vi "HFRR ADV v01.vi"() -> ()   [LabVIEW 2025] (continued)
                n2440 = local read "TEST STANDARD"() -> (w3160:T5)
                n2441 = Equal?(x=w3165, y=enum16{"ASTM D6079", "ISO 12156", "Custom"}."ISO 12156" ("Test Standard")) -> (x = y?=w3163:bool)
                n2442 = Equal?(x=w3160, y=enum16{"ASTM D6079", "ISO 12156", "Custom"}."ASTM D6079" ("Test Standard")) -> (x = y?=w3159:bool)
                n2443 = case shown="True" w3163 {
                  frame False {
                  }
                  frame True {
                    n2444 = local write "airtempflg"(FALSE ("airtempflg")) -> ()
                    n2445 = local write item#-1(TRUE ("Heater")) -> ()
                  }
                }
                n2446 = case shown="True" w3159 {
                  frame False {
                  }
                  frame True {
                    n2447 = local write "airtempflg"(TRUE ("airtempflg")) -> ()
                    n2448 = local write item#-1(FALSE ("Heater")) -> ()
                  }
                }
              }
            }
          }
          frame Enabled {
          }
        }
        n2449 = stacked-sequence {
          frame #0 {
            n2450 = case shown="True" "RST FF" {
              frame False {
              }
              frame True {
                w3179 = 0.0 ("X Scale.Range:Maximum")
                n2451 = property on="Frictional Force ( N )" class="WFChart (strict)"("XScale.Maximum"=600.0 ("X Scale.Range:Maximum"), "XScale.Minimum"=w3179, "YScale.Maximum"=10.0 ("Y Scale.Range:Maximum"), "YScale.Minimum"=w3179) -> ()  [unwired: 2 in, 2 out]
              }
            }
          }
          frame #1 {
            n2452 = case shown="True" "RST TEMP" {
              frame False {
              }
              frame True {
                n2453 = property on="Temperature ( Deg C )" class="WFChart (strict)"("XScale.Minimum"=0.0 ("X Scale.Range:Minimum"), "XScale.Maximum"=600.0 ("X Scale.Range:Maximum"), "YScale.Minimum"=0.0 ("Y Scale.Range:Minimum"), "YScale.Maximum"=100.0 ("Y Scale.Range:Maximum")) -> ()  [unwired: 2 in, 2 out]
              }
            }
          }
          frame #2 {
            n2454 = case shown="True" "RSTCOF" {
              frame False {
              }
              frame True {
                n2455 = property on="Coefficient of Friction" class="WFChart (strict)"("XScale.Minimum"=0.0 ("X Scale.Range:Minimum"), "XScale.Maximum"=600.0 ("X Scale.Range:Maximum"), "YScale.Maximum"=1.0 ("X Scale.Range:Minimum"), "YScale.Minimum"=0.0 ("X Scale.Range:Minimum")) -> ()  [unwired: 2 in, 2 out]
              }
            }
          }
          frame #3 {
            n2456 = case shown="True" "RSTCOF 2" {
              frame False {
              }
              frame True {
                (unwired) 100.0 ("Y Scale.Range:Maximum")
                (unwired) 0.0 ("Y Scale.Range:Minimum")
                (unwired) 600.0 ("X Scale.Range:Maximum")
                (unwired) 0.0 ("X Scale.Range:Minimum")
              }
            }
          }
          frame #4 {
            n2457 = case shown="True" "RSTCOF 3" {
              frame False {
              }
              frame True {
                n2458 = property on="Electrical Contact Resistance ( % )" class="WFChart (strict)"("XScale.Minimum"=0.0 ("X Scale.Range:Minimum"), "XScale.Maximum"=600.0 ("X Scale.Range:Maximum"), "YScale.Minimum"=0.0 ("Y Scale.Range:Minimum"), "YScale.Maximum"=100.0 ("Y Scale.Range:Maximum")) -> ()  [unwired: 2 in, 2 out]
              }
            }
          }
        }
        n2459 = local read "RUN"() -> (w3106:bool)
        n2460 = case shown="False" w3106 {
          frame False {
          }
          frame True {
          }
        }
        n2461 = local read "RUN"() -> (w3110:bool)
        n2462 = case shown="False" w3110 {
          tunnel: [FALSE ("TEST RUNNING") TRUE ("TEST RUNNING")] -> w3109
          frame False {
            w3198 = 0.0 ("Flag")
            n2463 = local write "Elapsed time"(0.0 ("elapsedtime")) -> ()
            n2464 = local write "Time Remaining"(w3198) -> ()
            n2465 = local write "Flag"(w3198) -> ()
            n2466 = local write "Remaining Time"(w3198) -> ()
          }
          frame True {
            n2467 = local write "Flag"(10.0 ("Flag")) -> ()
          }
        }
        n2468 = local read "AIR TEMP"() -> (w3104:dbl)
        n2469 = Greater Or Equal?(x=w3104, y=15.0) -> (x >= y?=w3105:bool)
        "powstat" <- w3105
        n2470 = case shown="True" "Save & Continue" {
          frame False {
          }
          frame True {
            n2471 = local read "USER ID"() -> (w3502:string)
            n2472 = local read "FILE"() -> (w3510:string)
            n2473 = String Length(string=w3510) -> (length=w3508:i32)
            n2474 = String Length(string=w3502) -> (length=w3505:i32)
            n2475 = Greater?(x=w3508, y=0) -> (0:w3507:bool)
            n2476 = Greater?(x=w3505, y=0) -> (0:w3504:bool)
            n2477 = And(x=w3507, y=w3504) -> (x .and. y?=w3503:bool)
            n2478 = case shown="True" w3503 {
              frame False {
                n2479 = stacked-sequence {
                  frame #0 {
                    n2480 = One Button Dialog(message="Please Enter a File Name and Operator ID to save data !", button name ("OK")="Ok") -> ()  [unwired: 1 out]
                  }
                  frame #1 {
                    n2481 = local write "Save & Continue"(FALSE ("OK Button")) -> ()
                  }
                }
                n2482 = local write "Save & Continue"(FALSE ("OK Button")) -> ()
              }
              frame True {
                n2483 = stacked-sequence {
                  frame #0 {
                    n2484 = local read "FILE"() -> (w3516:string)
                    n2485 = call "file check.vi"("file name in"=w3516) -> ("file name out"=w3515:string)  [unwired: 9 in, 1 out]
                    n2486 = call <vilib>:"Application Directory.vi"() -> ("Application Directory"=w3526:path)
                    n2487 = Build Path(base path=w3526, name or relative path="data") -> (appended path=w3525:path)
                    n2488 = call <vilib>:"Trim Whitespace.vi"("string"=w3515) -> ("trimmed string"=w3523:string)  [unwired: 1 in]
                    n2489 = call <vilib>:"Trim Whitespace.vi"("string"=w3515) -> ("trimmed string"=w3524:string)  [unwired: 1 in]
                    n2490 = List Folder(path=w3525) -> (folder names=w3521:string[])  [unwired: 3 in, 3 out]
                    n2491 = Match Pattern(string=w3523, regular expression="_(") -> (before substring=w3520:string)  [unwired: 1 in, 3 out]
                    n2492 = for {
                      tunnel: w3521 -> [w3535] mode=indexing
                      tunnel: w3520 -> [w3533]
                      shift-right: [w3531] -> w3518
                      shift-left: bool[] [] -> [w3532]
                      n2493 = Match Pattern(string=w3535, regular expression="_(") -> (before substring=w3534:string)  [unwired: 1 in, 3 out]
                      n2494 = Equal?(x=w3534, y=w3533) -> (x = y?=w3530:bool)
                      n2495 = case shown="True" w3530 {
                        tunnel: w3530 -> [_ w3538]
                        tunnel: w3532 -> [w3537 w3540]
                        tunnel: [w3537 w3539] -> w3531
                        frame False {
                        }
                        frame True {
                          n2496 = Insert Into Array(array=w3540, new element=w3538) -> (w3539:bool[])  [unwired: 1 in]
                        }
                      }
                    }
                    n2497 = Equal?(x=w3521, y=w3520) -> (x = y?=w3529:bool[])
                    n2498 = Or Array Elements(Boolean array=w3529) -> (logical OR=w3528:bool)
                    n2499 = Array Size(array=w3518) -> (size(s)=w3517:i32)
                    n2500 = case shown="True" w3528 {
                      tunnel: w3524 -> [_ w3548]
                      tunnel: w3517 -> [_ w3541]
                      frame False {
                      }
                      frame True {
                        n2501 = Number To Decimal String(number=w3541) -> (decimal integer string=w3544:string)  [unwired: 1 in]
                        n2502 = Search/Split String(string=w3548, search string/char (-)="_(" ("regular expression")) -> (substring before match=w3546:string)  [unwired: 1 in, 2 out]
                        n2503 = Concatenate Strings(w3546, "_(" ("regular expression"), w3544, ")" ("regular expression")) -> (w3542:string)
                        n2504 = local write "FILE"(w3542) -> ()
                      }
                    }
                  }
                  frame #1 {
                    w3551 = 0.0
                    w3564 = cluster{"y":dbl, dbl, "y":dbl}[] [] ("History Data")
                    w3565 = FALSE ("Heater Button")
                    (unwired) ")!" ("string")
                    (unwired) ")" ("string")
                    w3563 = dbl[] [] ("History Data")
                    w3569 = "\r"
                    # "C:\\WinDucom\\Data\\"
                    # "C:\\LAB-IQ-NXT\\data"
                    n2505 = local write "Humidity ( %RH )"(w3551) -> ()
                    n2506 = local write "Frequency ( Hz )"(w3551) -> ()
                    n2507 = local write "Stroke 3"(w3551) -> ()
                    n2508 = local write "speedop"(0.0 ("PIDclk 2")) -> ()
                    n2509 = local write "Set Temp 2"(65.0 ("Set Temp 2")) -> ()
                    n2510 = local write "AIR TEMP"(w3551) -> ()
                    n2511 = local write "clk"(0.0 ("clk")) -> ()
                    n2512 = local write "Stroke 4"(w3551) -> ()
                    n2513 = local write "COF 2"(w3551) -> ()
                    n2514 = local write "TEMP"(w3551) -> ()
                    n2515 = local write "ecr 3"(w3551) -> ()
                    n2516 = local write "FF 3"(w3551) -> ()
                    n2517 = local write "FF 2"(w3551) -> ()
                    n2518 = property on="Coefficient of Friction" class="WFChart (strict)"("History Data"=w3563) -> ()  [unwired: 2 in, 2 out]
                    n2519 = property on="Coefficient of Friction" class="WFChart (strict)"("History Data"=w3563) -> ()  [unwired: 2 in, 2 out]
                    n2520 = property on="Frictional Force ( N )" class="WFChart (strict)"("History Data"=w3563) -> ()  [unwired: 2 in, 2 out]
                    n2521 = property on="Electrical Contact Resistance ( % )" class="WFChart (strict)"("History Data"=w3563) -> ()  [unwired: 2 in, 2 out]
                    n2522 = property on="Electrical Contact Resistance ( % )" class="WFChart (strict)"("History Data"=w3563) -> ()  [unwired: 2 in, 2 out]
                    n2523 = property on="Temperature ( Deg C )" class="WFChart (strict)"("History Data"=w3563) -> ()  [unwired: 2 in, 2 out]
                    n2524 = property on="Frictional Force ( N )" class="WFChart (strict)"("History Data"=w3563) -> ()  [unwired: 2 in, 2 out]
                    n2525 = property on="Coefficient of Friction" class="WFChart (strict)"("History Data"=w3563) -> ()  [unwired: 2 in, 2 out]
                    n2526 = property on="Frictional Force ( N )" class="WFChart (strict)"("History Data"=w3563) -> ()  [unwired: 2 in, 2 out]
                    n2527 = property on="Electrical Contact Resistance ( % )" class="WFChart (strict)"("History Data"=w3563) -> ()  [unwired: 2 in, 2 out]
                    n2528 = property on="Temperature ( Deg C )" class="WFChart (strict)"("History Data"=w3563) -> ()  [unwired: 2 in, 2 out]
                    n2529 = property on="Stroke ( mm )" class="WFChart (strict)"("History Data"=w3564) -> ()  [unwired: 2 in, 2 out]
                    n2530 = property on="Stroke ( mm )" class="WFChart (strict)"("History Data"=w3564) -> ()  [unwired: 2 in, 2 out]
                    n2531 = local write "Humidity"(w3565) -> ()
                    n2532 = local write "Heater Button"(w3565) -> ()
                    n2533 = local read "FILE"() -> (w3559:string)
                    n2534 = disable-structure shown="Enabled" {
                      disable-tunnel: [w3603 _] -> w3550
                      frame Enabled {
                        n2535 = local read "NORMAL LOAD"() -> (w3603:dbl)
                      }
                      frame Disabled {
                      }
                    }
                    n2536 = call "file check.vi"("file name in"=w3559) -> ("error out"=w3562:errorcluster, "file name out"=w3556:string)  [unwired: 9 in]
                    n2537 = call "FILE PATH CREATION.vi"("error in"=w3562, "FILE NAME :"=w3556) -> ("FILE OUT"=w3555:path)  [unwired: 8 in, 1 out]
                    n2538 = Concatenate Strings(w3556, ".dgf" ("Substring")) -> (w3561:string)
                    n2539 = Concatenate Strings(w3556, ".duf" ("Substring")) -> (w3557:string)
                    n2540 = Multiply(x=w3550, y=1.0) -> (x*y=w3582:dbl)
                    n2541 = Build Path(base path=w3555, name or relative path=w3561) -> (appended path=w3554:path)
                    n2542 = Build Path(base path=w3555, name or relative path=w3557) -> (appended path=w3553:path)
                    n2543 = Number To Fractional String(number=w3582, width (-)=i16 5, precision (6)=i16 2) -> (F-format string=w3590:string)  [unwired: 1 in]
                    n2544 = local read "tested by"() -> (w3549:string)
                    n2545 = local read "Fuel Discription :"() -> (w3578:string)
                    n2546 = local read "Batch Ref Num :"() -> (w3567:string)
                    n2547 = Get Date/Time String(date format (0)=enum16{"short", "long", "abbreviated"}."short") -> (date string=w3601:string, time string=w3598:string)  [unwired: 2 in]
                    n2548 = local read "Remarks :"() -> (w3577:string)
                    n2549 = Concatenate Strings("Load :- " ("Substring"), w3590, " grams ," ("Substring")) -> (w3589:string)
                    n2550 = local read "String 41"() -> (w3570:string)
                    n2551 = Concatenate Strings(w3578) -> (w3579:string)
                    n2552 = Concatenate Strings(w3567) -> (w3566:string)
                    n2553 = Concatenate Strings(w3549) -> (w3573:string)
                    n2554 = Concatenate Strings("(" ("Substring"), w3601, ")" ("Substring"), w3598) -> (w3572:string)
                    "concatenated string" <- w3572
                    n2555 = Concatenate Strings(w3577, "," ("string")) -> (w3576:string)
                    n2556 = Concatenate Strings("  TIME;      COF;       STROKE;     AIR TEMP;  TEMP;  HUMIDITY;  ECR; PID-OUT; FREQUENCY" ("Substring"), "\r") -> (w3585:string)
                    n2557 = Concatenate Strings(w3570, w3569, "Fuel Discription :-" ("Substring"), w3579, w3569, w3589, w3569, "Batch Ref Num :-" ("Substring"), w3566, w3569, " Remarks :- " ("Substring"), w3576, w3569, " Date :- " ("Substring"), w3572, w3569, "Tested By :-" ("Substring"), w3573) -> (w3583:string)
                    "REMARKS" <- w3583
                    n2558 = call <vilib>:"Write Characters To File.vi"("append to file? (new file:F)"=FALSE, "character string"=w3585, "file path (dialog if empty)"=w3554) -> ()  [unwired: 2 in, 1 out]
                    n2559 = call <vilib>:"Write Characters To File.vi"("append to file? (new file:F)"=FALSE, "character string"=w3583, "file path (dialog if empty)"=w3553) -> ()  [unwired: 2 in, 1 out]
                  }
                  frame #2 {
                    n2560 = local write "Cycles elapsed"(0 ("Cycles elapsed")) -> ()
                    n2561 = local write "cyclecount"(0 ("cyclecount")) -> ()
                    n2562 = local write "Save & Continue"(FALSE ("OK")) -> ()
                    n2563 = local write "autostrtflg"(TRUE ("autostrtflg")) -> ()
                    n2564 = local write "Save"(FALSE ("Save")) -> ()
                    n2565 = Get Date/Time In Seconds() -> (seconds since 1Jan1904=w3608:timestamp)
                    n2566 = To Double Precision Float(number=w3608) -> (double precision float=w3607:dbl)
                    n2567 = local write "acq timer"(w3607) -> ()
                    n2568 = One Button Dialog(message="Please ensure sample is mounted properly and machine is ready in all aspects for testing !", button name ("OK")="Ok") -> ()  [unwired: 1 out]
                  }
                  frame #3 {
                    n2569 = stacked-sequence {
                      frame #0 {
                        n2570 = local write "Main Dashboard Buttons"(T1."Dashboard" ("Main Dashboard Buttons")) -> ()
                        n2571 = local write "Main Tab"(T4."Acquire" ("Main Tab")) -> ()
                      }
                      frame #1 {
                        n2572 = local write "EVENT LOG"("" ("EVENT LOG")) -> ()
                      }
                      frame #2 {
                        n2573 = Wait (ms)(milliseconds to wait=u32 50) -> ()  [unwired: 1 out]
                      }
                      frame #3 {
                        n2574 = disable-structure shown="Disabled" {
                          frame Disabled {
                            n2575 = local read "EVENT LOG"() -> (w3620:string)
                            n2576 = call "Event Log.vi"("Content"="Test Details", "EVENT LOG"=w3620) -> ("EVENT LOG"=w3619:string)  [unwired: 8 in, 1 out]
                            n2577 = local write "EVENT LOG"(w3619) -> ()
                          }
                          frame Enabled {
                          }
                        }
                      }
                      frame #4 {
                        n2578 = Wait (ms)(milliseconds to wait=u32 50) -> ()  [unwired: 1 out]
                      }
                      frame #5 {
                        n2579 = local read "FILE"() -> (w3622:string)
                        n2580 = Concatenate Strings("File Name :" ("Content"), w3622) -> (w3623:string)
                        n2581 = local read "EVENT LOG"() -> (w3626:string)
                        n2582 = call "Event Log.vi"("Content"=w3623, "EVENT LOG"=w3626) -> ("EVENT LOG"=w3625:string)  [unwired: 8 in, 1 out]
                        n2583 = local write "EVENT LOG"(w3625) -> ()
                      }
                      frame #6 {
                        n2584 = Wait (ms)(milliseconds to wait=u32 50) -> ()  [unwired: 1 out]
                      }
                      frame #7 {
                        n2585 = local read "Batch Ref Num :"() -> (w3628:string)
                        n2586 = Concatenate Strings("Batch Ref No :" ("Content"), w3628) -> (w3629:string)
                        n2587 = local read "EVENT LOG"() -> (w3632:string)
                        n2588 = call "Event Log.vi"("Content"=w3629, "EVENT LOG"=w3632) -> ("EVENT LOG"=w3631:string)  [unwired: 8 in, 1 out]
                        n2589 = local write "EVENT LOG"(w3631) -> ()
                      }
                      frame #8 {
                        n2590 = Wait (ms)(milliseconds to wait=u32 50) -> ()  [unwired: 1 out]
                      }
                      frame #9 {
                        n2591 = local read "tested by"() -> (w3634:string)
                        n2592 = Concatenate Strings("Tested By :" ("Content"), w3634) -> (w3635:string)
                        n2593 = local read "EVENT LOG"() -> (w3638:string)
                        n2594 = call "Event Log.vi"("Content"=w3635, "EVENT LOG"=w3638) -> ("EVENT LOG"=w3637:string)  [unwired: 8 in, 1 out]
                        n2595 = local write "EVENT LOG"(w3637) -> ()
                      }
                      frame #10 {
                        n2596 = Wait (ms)(milliseconds to wait=u32 50) -> ()  [unwired: 1 out]
                      }
                      frame #11 {
                        n2597 = local read "TEST STANDARD"() -> (w3641:T5)
                        n2598 = case shown="\"ASTM D6079\", Default" w3641 {
                          tunnel: ["ASTM D6079" "ISO 12156" "CEC F-096-A-06" "Custom"] -> w3640
                          frame "ASTM D6079", Default {
                          }
                          frame "ISO 12156" {
                          }
                          frame "CEC F-096-A-06" {
                          }
                          frame "Custom" {
                          }
                        }
                        n2599 = Concatenate Strings("Test Standard :" ("Content"), w3640) -> (w3642:string)
                        n2600 = local read "EVENT LOG"() -> (w3645:string)
                        n2601 = call "Event Log.vi"("Content"=w3642, "EVENT LOG"=w3645) -> ("EVENT LOG"=w3644:string)  [unwired: 8 in, 1 out]
                        n2602 = local write "EVENT LOG"(w3644) -> ()
                      }
                      frame #12 {
                        n2603 = Wait (ms)(milliseconds to wait=u32 50) -> ()  [unwired: 1 out]
                      }
                      frame #13 {
                        n2604 = local read "Fuel Discription :"() -> (w3651:string)
                        n2605 = Concatenate Strings("Fuel Description :" ("Content"), w3651) -> (w3652:string)
                        n2606 = local read "EVENT LOG"() -> (w3655:string)
                        n2607 = call "Event Log.vi"("Content"=w3652, "EVENT LOG"=w3655) -> ("EVENT LOG"=w3654:string)  [unwired: 8 in, 1 out]
                        n2608 = local write "EVENT LOG"(w3654) -> ()
                      }
                      frame #14 {
                        n2609 = Wait (ms)(milliseconds to wait=u32 50) -> ()  [unwired: 1 out]
                      }
                      frame #15 {
                        n2610 = local read "Remarks :"() -> (w3657:string)
                        n2611 = Concatenate Strings("Remarks :" ("Content"), w3657) -> (w3658:string)
                        n2612 = local read "EVENT LOG"() -> (w3661:string)
                        n2613 = call "Event Log.vi"("Content"=w3658, "EVENT LOG"=w3661) -> ("EVENT LOG"=w3660:string)  [unwired: 8 in, 1 out]
                        n2614 = local write "EVENT LOG"(w3660) -> ()
                      }
                      frame #16 {
                        n2615 = Wait (ms)(milliseconds to wait=u32 50) -> ()  [unwired: 1 out]
                      }
                      frame #17 {
                        n2616 = local read "USER ID"() -> (w3663:string)
                        n2617 = Concatenate Strings("Operator ID :" ("Content"), w3663) -> (w3665:string)
                        n2618 = local read "EVENT LOG"() -> (w3667:string)
                        n2619 = call "Event Log.vi"("Content"=w3665, "EVENT LOG"=w3667) -> ("EVENT LOG"=w3666:string)  [unwired: 8 in, 1 out]
                        n2620 = local write "EVENT LOG"(w3666) -> ()
                      }
                      frame #18 {
                        n2621 = Wait (ms)(milliseconds to wait=u32 50) -> ()  [unwired: 1 out]
                      }
                      frame #19 {
                        n2622 = disable-structure shown="Disabled" {
                          frame Disabled {
                            n2623 = local read "EVENT LOG"() -> (w3671:string)
                            n2624 = call "Event Log.vi"("Content"="Test Parameter", "EVENT LOG"=w3671) -> ("EVENT LOG"=w3670:string)  [unwired: 8 in, 1 out]
                            n2625 = local write "EVENT LOG"(w3670) -> ()
                          }
                          frame Enabled {
                          }
                        }
                      }
                      frame #20 {
                        n2626 = Wait (ms)(milliseconds to wait=u32 50) -> ()  [unwired: 1 out]
                      }
                      frame #21 {
                        n2627 = local read "Set Hz"() -> (w3675:dbl)
                        n2628 = Number To Fractional String(number=w3675, precision (6)=i16 2) -> (F-format string=w3674:string)  [unwired: 2 in]
                        n2629 = Concatenate Strings("Set Frequency [Hz] :" ("Content"), w3674) -> (w3677:string)
                        n2630 = local read "EVENT LOG"() -> (w3679:string)
                        n2631 = call "Event Log.vi"("Content"=w3677, "EVENT LOG"=w3679) -> ("EVENT LOG"=w3678:string)  [unwired: 8 in, 1 out]
                        n2632 = local write "EVENT LOG"(w3678) -> ()
                      }
                      frame #22 {
                        n2633 = Wait (ms)(milliseconds to wait=u32 50) -> ()  [unwired: 1 out]
                      }
                      frame #23 {
                        n2634 = local read "NORMAL LOAD"() -> (w3682:dbl)
                        n2635 = Number To Fractional String(number=w3682, precision (6)=i16 2) -> (F-format string=w3683:string)  [unwired: 2 in]
                        n2636 = Concatenate Strings("Applied Load [grams] :" ("Content"), w3683) -> (w3685:string)
                        n2637 = local read "EVENT LOG"() -> (w3687:string)
                        n2638 = call "Event Log.vi"("Content"=w3685, "EVENT LOG"=w3687) -> ("EVENT LOG"=w3686:string)  [unwired: 8 in, 1 out]
                        n2639 = local write "EVENT LOG"(w3686) -> ()
                      }
                      frame #24 {
                        n2640 = Wait (ms)(milliseconds to wait=u32 50) -> ()  [unwired: 1 out]
                      }
                      frame #25 {
                        n2641 = local read "Set Strk"() -> (w3690:dbl)
                        n2642 = Number To Fractional String(number=w3690, precision (6)=i16 2) -> (F-format string=w3691:string)  [unwired: 2 in]
                        n2643 = Concatenate Strings("Set Stroke [mm] :" ("Content"), w3691) -> (w3693:string)
                        n2644 = local read "EVENT LOG"() -> (w3695:string)
                        n2645 = call "Event Log.vi"("Content"=w3693, "EVENT LOG"=w3695) -> ("EVENT LOG"=w3694:string)  [unwired: 8 in, 1 out]
                        n2646 = local write "EVENT LOG"(w3694) -> ()
                      }
                      frame #26 {
                        n2647 = Wait (ms)(milliseconds to wait=u32 50) -> ()  [unwired: 1 out]
                      }
                      frame #27 {
                        n2648 = local read "Set Temp"() -> (w3698:dbl)
                        n2649 = Number To Fractional String(number=w3698, precision (6)=i16 2) -> (F-format string=w3699:string)  [unwired: 2 in]
                        n2650 = Concatenate Strings("Set Temperature [deg C] :" ("Content"), w3699) -> (w3701:string)
                        n2651 = local read "EVENT LOG"() -> (w3703:string)
                        n2652 = call "Event Log.vi"("Content"=w3701, "EVENT LOG"=w3703) -> ("EVENT LOG"=w3702:string)  [unwired: 8 in, 1 out]
                        n2653 = local write "EVENT LOG"(w3702) -> ()
                      }
                      frame #28 {
                        n2654 = Wait (ms)(milliseconds to wait=u32 50) -> ()  [unwired: 1 out]
                      }
                      frame #29 {
                        n2655 = local read "Set Rh"() -> (w3706:dbl)
                        n2656 = Number To Fractional String(number=w3706, precision (6)=i16 2) -> (F-format string=w3707:string)  [unwired: 2 in]
                        n2657 = Concatenate Strings("Set Humidity [%RH] :" ("Content"), w3707) -> (w3709:string)
                        n2658 = local read "EVENT LOG"() -> (w3711:string)
                        n2659 = call "Event Log.vi"("Content"=w3709, "EVENT LOG"=w3711) -> ("EVENT LOG"=w3710:string)  [unwired: 8 in, 1 out]
                        n2660 = local write "EVENT LOG"(w3710) -> ()
                      }
                      frame #30 {
                        n2661 = Wait (ms)(milliseconds to wait=u32 50) -> ()  [unwired: 1 out]
                      }
                      frame #31 {
                        n2662 = local read "test time"() -> (w3714:dbl)
                        n2663 = Number To Fractional String(number=w3714, precision (6)=i16 1) -> (F-format string=w3715:string)  [unwired: 2 in]
                        n2664 = Concatenate Strings("Test Duration [mins] :" ("Content"), w3715) -> (w3717:string)
                        n2665 = local read "EVENT LOG"() -> (w3719:string)
                        n2666 = call "Event Log.vi"("Content"=w3717, "EVENT LOG"=w3719) -> ("EVENT LOG"=w3718:string)  [unwired: 8 in, 1 out]
                        n2667 = local write "EVENT LOG"(w3718) -> ()
                      }
                      frame #32 {
                        w3720 = dbl[] [] ("History Data")
                        w3721 = cluster{"y":dbl, dbl, "y":dbl}[] [] ("History Data")
                        w3722 = FALSE ("Visible")
                        n2668 = property on="Stroke ( mm )" class="WFChart (strict)"("History Data"=w3721) -> ()  [unwired: 2 in, 2 out]
                        n2669 = property on="Temperature ( Deg C )" class="WFChart (strict)"("History Data"=w3720) -> ()  [unwired: 2 in, 2 out]
                        n2670 = property on="Electrical Contact Resistance ( % )" class="WFChart (strict)"("History Data"=w3720) -> ()  [unwired: 2 in, 2 out]
                        n2671 = property on="Coefficient of Friction" class="WFChart (strict)"("History Data"=w3720) -> ()  [unwired: 2 in, 2 out]
                        n2672 = property on="Frictional Force ( N )" class="WFChart (strict)"("History Data"=w3720) -> ()  [unwired: 2 in, 2 out]
                        n2673 = property on="Coefficient of Friction" class="WFChart (strict)"("History Data"=w3720) -> ()  [unwired: 2 in, 2 out]
                        n2674 = property on="Frictional Force ( N )" class="WFChart (strict)"("History Data"=w3720) -> ()  [unwired: 2 in, 2 out]
                        n2675 = property on="Electrical Contact Resistance ( % )" class="WFChart (strict)"("History Data"=w3720) -> ()  [unwired: 2 in, 2 out]
                        n2676 = property on="Stroke ( mm )" class="WFChart (strict)"("History Data"=w3721) -> ()  [unwired: 2 in, 2 out]
                        n2677 = property on="Temperature ( Deg C )" class="WFChart (strict)"("History Data"=w3720) -> ()  [unwired: 2 in, 2 out]
                        n2678 = property on="Service Password Log" class="Str"("Visible"=w3722) -> ()  [unwired: 2 in, 2 out]
                        n2679 = property on="Password 3" class="Clust (strict)"("Visible"=w3722) -> ()  [unwired: 2 in, 2 out]
                      }
                    }
                    "TEST FILE NAM,E SAVED" <- TRUE ("TEST FILE NAM,E SAVED")
                  }
                }
              }
            }
          }
        }
        n2680 = local write "Test \nStatus"(w3109) -> ()
        n2681 = local write "Save"(w3109) -> ()
        n2682 = local read "Main Tab"() -> (w3103:T4)
        n2683 = case shown="True" w3106 {
          frame False {
            n2684 = local read "Rt 3"() -> (w3170:bool)
            n2685 = case shown="True" w3170 {
              frame False {
              }
              frame True {
                n2686 = local write "Rt 3"(FALSE ("Rt 3")) -> ()
              }
            }
            "Rt" <- TRUE ("Rt")
            "Rt 2" <- FALSE ("Rt")
          }
          frame True {
            n2687 = local read "Rt"() -> (w3176:bool)
            n2688 = local write "Rt 2"(TRUE ("Rt 2")) -> ()
            n2689 = case shown="True" w3176 {
              frame False {
              }
              frame True {
                n2690 = local write "Rt"(FALSE ("Rt")) -> ()
              }
            }
            "Rt 3" <- TRUE ("Rt 3")
          }
        }
        n2691 = case shown="\"Acquire\"" w3103 {
          tunnel: w3105 -> [_ w3205]
          frame Default {
            w3204 = 0.0 ("output")
            n2692 = local write "PID-out"(w3204) -> ()
            n2693 = local write "Frequency ( Hz )"(w3204) -> ()
            n2694 = local write "STROKE Initialize"(TRUE ("STROKE Initialize")) -> ()
          }
          frame "Acquire" {
            n2695 = stacked-sequence {
              frame #0 {
                n2696 = local read "Auto Start Test"() -> (w3207:bool)
                n2697 = case shown="True" w3207 {
                  tunnel: "RUN" -> [w3228 w3231]
                  tunnel: [w3228 w3230] -> w3208
                  frame False {
                  }
                  frame True {
                    n2698 = local read "Auto Start Temp"() -> (w3229:bool)
                    n2699 = Or(x=w3231, y=w3229) -> (x .or. y?=w3230:bool)
                  }
                }
                n2700 = local read "clk"() -> (w3227:dbl)
                n2701 = local read "Save"() -> (w3223:bool)
                n2702 = Equal?(x=w3227, y=0.0) -> (x = y?=w3224:bool)
                n2703 = And(x=w3224, y=w3223) -> (x .and. y?=w3225:bool)
                n2704 = Not(x="Engage") -> (.not. x?=w3214:bool)
                n2705 = case shown="False" w3208 {
                  tunnel: [0.0 w3255] -> w3210
                  frame False {
                    (unwired) TRUE ("Visible")
                    n2706 = local read "Auto Start Test"() -> (w3235:bool)
                    n2707 = local write "Start Time"(TRUE ("Start Time")) -> ()
                    n2708 = property on="Stroke 2" class="DigNum (strict)"("Visible"=FALSE) -> ()  [unwired: 2 in, 2 out]
                    n2709 = case shown="False" w3235 {
                      frame False {
                        n2710 = property on="Heater Button" class="Bool (strict)"("DisabledEnum"=T19."Enabled" ("Disabled")) -> ()  [unwired: 2 in, 2 out]
                        n2711 = property on="Humidity" class="Bool (strict)"("DisabledEnum"=T19."Enabled" ("Disabled")) -> ()  [unwired: 2 in, 2 out]
                      }
                      frame True {
                      }
                    }
                    n2712 = case shown="False" "TestCompFlg" {
                      frame False {
                        n2713 = local read "StartFlg"() -> (w3243:bool)
                        n2714 = case shown="True" w3243 {
                          frame False {
                          }
                          frame True {
                            n2715 = stacked-sequence {
                              frame #0 {
                                n2716 = local read "EVENT LOG"() -> (w3247:string)
                                n2717 = call "Event Log.vi"("Content"="Test was interrupted", "EVENT LOG"=w3247) -> ("EVENT LOG"=w3248:string)  [unwired: 8 in, 1 out]
                                n2718 = local write "EVENT LOG"(w3248) -> ()
                                n2719 = property on="RUN" class="Bool (strict)"("Visible"=TRUE) -> ()  [unwired: 2 in, 2 out]
                                n2720 = property on="Auto Start Test" class="Bool (strict)"("Visible"=TRUE) -> ()  [unwired: 2 in, 2 out]
                              }
                              frame #1 {
                                w3251 = FALSE ("StartFlg")
                                n2721 = property on="Heater Button" class="Bool (strict)"("Val(Sgnl)"=FALSE ("Value (Signaling)")) -> ()  [unwired: 2 in, 2 out]
                                n2722 = local write "Heater Button"(w3251) -> ()
                                n2723 = local write "StartFlg"(w3251) -> ()
                                n2724 = local write "Humidity"(w3251) -> ()
                                n2725 = local write "Humidity 2"(TRUE ("Humidity")) -> ()
                              }
                              frame #2 {
                                n2726 = local write "Due Write"("VC;0" ("Command")) -> ()
                              }
                              frame #3 {
                                n2727 = Wait (ms)(milliseconds to wait=u32 1500) -> ()  [unwired: 1 out]
                              }
                              frame #4 {
                                n2728 = local write "Due Write"("HE;0" ("Command")) -> ()
                              }
                            }
                          }
                        }
                      }
                      frame True {
                      }
                    }
                    n2729 = local write "String 14"("Test will autostart once parameters reach the set value." ("String 14")) -> ()
                  }
                  frame True {
                    (unwired) FALSE ("Visible")
                    n2730 = property on="Stroke 2" class="DigNum (strict)"("Visible"=TRUE) -> ()  [unwired: 2 in, 2 out]
                    n2731 = property on="STOP 2" class="Bool (strict)"("Disabled"=u8 2) -> ()  [unwired: 2 in, 2 out]
                    n2732 = local write "String 14"(" Running....." ("String 14")) -> ()
                    n2733 = property on="Heater Button" class="Bool (strict)"("DisabledEnum"=T19."Disabled and Grayed Out" ("Disabled")) -> ()  [unwired: 2 in, 2 out]
                    n2734 = property on="Humidity" class="Bool (strict)"("DisabledEnum"=T19."Disabled and Grayed Out" ("Disabled")) -> ()  [unwired: 2 in, 2 out]
                    n2735 = case shown="True" "Start Time" {
                      selector: "Start Time" -> [_ w3274]
                      frame False {
                      }
                      frame True {
                        n2736 = Not(x=w3274) -> (.not. x?=w3273:bool)
                        n2737 = local write "Start Time"(w3273) -> ()
                        n2738 = local read "EVENT LOG"() -> (w3275:string)
                        n2739 = call "Event Log.vi"("Content"="Test in progress", "EVENT LOG"=w3275) -> ("EVENT LOG"=w3277:string)  [unwired: 8 in, 1 out]
                        n2740 = local write "EVENT LOG"(w3277) -> ()
                      }
                    }
                    n2741 = disable-structure shown="Enabled" {
                      disable-tunnel: [w3266 w3272] -> w3255
                      frame Disabled {
                        n2742 = local read "Set Hz"() -> (w3269:dbl)
                        n2743 = call <vilib>:"Uniform White Noise Waveform.vi"() -> ("signal out"=w3268:waveform(dbl))  [unwired: 10 in, 1 out]
                        n2744 = Random Number (0-1)() -> (number: 0 to 1=w3265:dbl)
                        n2745 = Add(x=w3269, y=w3268) -> (x+y=w3267:waveform(dbl))
                        n2746 = Multiply(x=ext 0.01 ("y"), y=w3265) -> (x*y=w3263:ext)
                        n2747 = Multiply(x=w3267, y=w3263) -> (x*y=w3266:waveform(ext))
                      }
                      frame Enabled {
                        n2748 = call-poly <vilib>:"Random Number (Range).vi"("lower bound (0)"=49.89, "upper bound (100)"=50.8) -> ("number"=w3272:dbl)  [unwired: 9 in]
                      }
                    }
                    "StartFlg" <- TRUE ("StartFlg")
                  }
                }
                n2749 = case shown="True" w3225 {
                  frame False {
                  }
                  frame True {
                    n2750 = local write "clk"(10.0 ("clk")) -> ()
                    n2751 = Get Date/Time In Seconds() -> (seconds since 1Jan1904=w3280:timestamp)
                    n2752 = To Double Precision Float(number=w3280) -> (double precision float=w3278:dbl)
                    n2753 = local write "acq timer"(w3278) -> ()
                    n2754 = local write "act save time"(w3278) -> ()
                  }
                }
                n2755 = call "Elapsed Time"("Time Target (s)"="Countdown", "Reset"=w3214) -> ("Elapsed Time (s)"=w3219:dbl, "Time has Elapsed"=w3217:bool)  [unwired: 10 in, 6 out]
                "Countdown 2" <- w3219
                n2756 = Subtract(x=w3219, y=2.0) -> (x-y=w3222:dbl)
                n2757 = Less?(x=w3222, y="Countdown") -> (x < y?=w3220:bool)
                n2758 = And(x=w3220, y=w3217) -> (x .and. y?=w3216:bool)
                n2759 = case shown="True" w3216 {
                  frame False {
                  }
                  frame True {
                    (unwired) dbl[] [] ("History Data")
                    n2760 = local write "Engage"(FALSE ("Engage")) -> ()
                    n2761 = local write "RUN"(TRUE ("RUN")) -> ()
                    n2762 = local read "Humidity ( %RH )"() -> (→"Rh Before":dbl)
                  }
                }
                n2763 = local read "Test \nStatus"() -> (w3212:bool)
                n2764 = Select(t=w3210, s=w3212, f=0.0) -> (s? t:f=w3211:dbl)
                n2765 = local write "Frequency ( Hz )"(w3211) -> ()
              }
              frame #1 {
                w3303 = 1000000.0 ("x")
                # "HC;1/0\nST;VALUE"
                # "Elapsed time\ncof\nstroke\nAir temp\nTemp\nHumidity"
                # "acq timer\n\nact save time"
                # "convert to microseconds"
                n2766 = local read "COUNT"() -> (w3286:i32)
                n2767 = local read "Rate"() -> (w3299:dbl)
                n2768 = Divide(x=w3303, y=w3299) -> (x/y=w3304:dbl)
                n2769 = Greater Or Equal?(x=w3286, y=250) -> (x >= y?=w3285:bool)
                n2770 = Get Date/Time In Seconds() -> (seconds since 1Jan1904=w3306:timestamp)
                n2771 = case shown="True" w3285 {
                  frame False {
                    n2772 = local read "COUNT"() -> (w3307:i32)
                    n2773 = Increment(x=w3307) -> (x+1=w3308:i32)
                    n2774 = local write "COUNT"(w3308) -> ()
                  }
                  frame True {
                    n2775 = local write "COUNT"(0 ("COUNT")) -> ()
                  }
                }
                n2776 = local read "Samplingtime 2"() -> (w3284:dbl)
                n2777 = local read "act save time"() -> (w3301:dbl)
                n2778 = Divide(x=w3304, y=w3303) -> (x/y=w3302:dbl)
                n2779 = To Double Precision Float(number=w3306) -> (double precision float=w3295:dbl)
                n2780 = Add(x=w3301, y=w3284) -> (x+y=w3300:dbl)
                n2781 = local read "acq timer"() -> (w3305:dbl)
                n2782 = local read "COUNT"() -> (w3288:i32)
                n2783 = Greater Or Equal?(x=w3295, y=w3300) -> (x >= y?=w3283:bool)
                n2784 = Multiply(x=w3302, y=w3288) -> (x*y=w3294:dbl)
                n2785 = Subtract(x=w3295, y=w3305) -> (x-y=w3297:dbl)
                n2786 = local read "Save"() -> (w3298:bool)
                n2787 = Add(x=w3297, y=w3294) -> (x+y=w3281:dbl)
                "Elapsed time 3" <- w3281
                n2788 = And(x=w3283, y=w3298) -> (x .and. y?=w3296:bool)
                n2789 = Divide(x=w3281, y=60.0) -> (x/y=w3292:dbl)
                n2790 = local read "Test \nStatus"() -> (w3282:bool)
                n2791 = local read "clk"() -> (w3289:dbl)
                n2792 = Equal?(x=w3289, y=10.0) -> (x = y?=w3291:bool)
                n2793 = case shown="True" w3296 {
                  tunnel: w3295 -> [_ w3422]
                  tunnel: [FALSE ("Boolean 2") TRUE ("Boolean 2")] -> _
                  frame False {
                  }
                  frame True {
                    w3376 = ";" ("Substring")
                    # "Pid out/\nFreq response value"
                    n2794 = local write "act save time"(w3422) -> ()
                    n2795 = local read "FILE"() -> (w3370:string)
                    n2796 = call "file check.vi"("file name in"=w3370) -> ("error out"=w3373:errorcluster, "file name out"=w3368:string)  [unwired: 9 in]
                    n2797 = local read "LVDT STROKE"() -> (w3365:dbl)
                    n2798 = local read "Add up Stroke"() -> (w3363:dbl)
                    n2799 = call "FILE PATH CREATION.vi"("error in"=w3373, "FILE NAME :"=w3368) -> ("FILE OUT"=w3371:path)  [unwired: 8 in, 1 out]
                    n2800 = local read "STROKE Initialize"() -> (w3358:bool)
                    n2801 = Concatenate Strings(w3368, ".dgf" ("Substring")) -> (w3372:string)
                    n2802 = Subtract(x=w3365, y=w3363) -> (x-y=w3364:dbl)
                    n2803 = Absolute Value(x=w3364) -> (abs(x)=w3361:dbl)
                    n2804 = local read "FF 2"() -> (→"Frictional Force ( N )" →"Frictional Force ( N )":dbl)
                    n2805 = Build Path(base path=w3371, name or relative path=w3372) -> (appended path=w3367:path)
                    n2806 = flat-sequence {
                      tunnel: w3361 -> [w3427]
                      tunnel: [w3426] -> w3359
                      tunnel: w3358 -> [w3424]
                      tunnel: [w3429] -> w3360
                      tunnel: w3359 -> [w3429]
                      frame #0 {
                        n2807 = call <vilib>:"Mean PtByPt.vi"("x"=w3427, "sample length"="STROKE FILTER", "initialize"=w3424) -> ("mean"=w3426:dbl)  [unwired: 1 in, 1 out]
                      }
                      frame #1 {
                        "STROKE Initialize" <- FALSE ("STROKE Initialize")
                      }
                    }
                    n2808 = local read "COF 2"() -> (w3381:dbl)
                    "Coefficient of Friction" <- w3381
                    "COF 4" <- w3381
                    "Coefficient of Friction" <- w3381
                    n2809 = local read "TEMP"() -> (w3384:dbl)
                    "Temperature ( Deg C )" <- w3384
                    n2810 = local read "Humidity ( %RH )"() -> (w3383:dbl)
                    n2811 = local read "Frequency ( Hz )"() -> (w3390:dbl)
                    n2812 = local read "LVDT STROKE DISPLAY"() -> (w3362:dbl)
                    n2813 = local read "Elapsed time"() -> (w3415:dbl)
                    n2814 = local read "AIR TEMP"() -> (w3388:dbl)
                    n2815 = local read "PID-out"() -> (w3393:dbl)
                    n2816 = local write "Temperature ( Deg C )"(w3384) -> ()
                    n2817 = Number To Fractional String(number=w3362, width (-)=i16 9 ("precision (6)"), precision (6)=i16 6) -> (F-format string=w3408:string)  [unwired: 1 in]
                    n2818 = Number To Fractional String(number=w3388, width (-)=i16 9 ("precision (6)"), precision (6)=i16 3) -> (F-format string=w3407:string)  [unwired: 1 in]
                    n2819 = Number To Fractional String(number=w3384, width (-)=i16 9 ("precision (6)"), precision (6)=i16 3) -> (F-format string=w3404:string)  [unwired: 1 in]
                    n2820 = Number To Fractional String(number=w3383, width (-)=i16 9 ("precision (6)"), precision (6)=i16 3) -> (F-format string=w3401:string)  [unwired: 1 in]
                    n2821 = Number To Fractional String(number=0.0, width (-)=i16 9 ("precision (6)"), precision (6)=i16 3) -> (F-format string=w3398:string)  [unwired: 1 in]
                    n2822 = Number To Fractional String(number=w3393, width (-)=i16 9 ("precision (6)"), precision (6)=i16 3) -> (F-format string=w3394:string)  [unwired: 1 in]
                    n2823 = Number To Fractional String(number=w3390, width (-)=i16 9 ("precision (6)"), precision (6)=i16 3) -> (F-format string=w3389:string)  [unwired: 1 in]
                    n2824 = Number To Fractional String(number=w3381, width (-)=i16 9 ("precision (6)"), precision (6)=i16 6) -> (F-format string=w3416:string)  [unwired: 1 in]
                    n2825 = Number To Fractional String(number=w3415, width (-)=i16 14 ("precision (6)"), precision (6)=i16 3) -> (F-format string=w3417:string)  [unwired: 1 in]
                    n2826 = Bundle("y"=1.02, "LVDT STROKE DISPLAY"=w3362, "y"=0.98) -> (w3382:T30)  [unwired: 1 in]
                    n2827 = Number To Fractional String(number="Ambient Humidity :", width (-)=i16 9 ("precision (6)"), precision (6)=i16 6) -> (F-format string=w3374:string)  [unwired: 1 in]
                    n2828 = local read "RUN"() -> (w3380:bool)
                    n2829 = case shown="True" w3380 {
                      tunnel: w3382 -> [_ w3433]
                      tunnel: w3362 -> [_ w3432]
                      tunnel: w3362 -> [_ w3430]
                      tunnel: w3362 -> [_ w3431]
                      frame False {
                      }
                      frame True {
                        "Stroke ( mm )" <- w3433
                        "Stroke ( mm )" <- w3433
                        "Stroke 4" <- w3432
                        "Stroke 3" <- w3430
                        "Stroke 2" <- w3431
                        "measured_stroke" <- w3430
                      }
                    }
                    n2830 = Concatenate Strings(w3417, w3376, w3416, w3376, w3408, w3376, w3407, w3376, w3404, w3376, w3401, w3376, w3398, w3376, w3394, w3376, w3389, w3376, w3374, "\r") -> (w3414:string)
                    n2831 = call <vilib>:"Write Characters To File.vi"("append to file? (new file:F)"=TRUE, "character string"=w3414, "file path (dialog if empty)"=w3367) -> ()  [unwired: 2 in, 1 out]
                    "refresh flag" <- TRUE ("refresh flag")
                    "LVDT STROKE Actual" <- w3360
                  }
                }
                n2832 = case shown="True" w3282 {
                  tunnel: w3292 -> [_ w3318]
                  tunnel: w3297 -> [_ w3328]
                  tunnel: [0.0 w3324] -> _
                  tunnel: w3291 -> [_ w3323]
                  tunnel: [0.0 w3322] -> _
                  tunnel: w3281 -> [_ w3322]
                  tunnel: w3295 -> [w3311 _]
                  frame False {
                    n2833 = local write "acq timer"(w3311) -> ()
                    n2834 = local write "Test Duration Status"(0.0 ("Test Duration Status")) -> ()
                  }
                  frame True {
                    n2835 = local read "Set Hz"() -> (w3325:dbl)
                    n2836 = local write "Elapsed time"(w3318) -> ()
                    n2837 = local read "test time"() -> (w3317:dbl)
                    n2838 = Multiply(x=w3328, y=w3325) -> (x*y=w3327:dbl)
                    n2839 = case shown="False" w3323 {
                      tunnel: w3327 -> [w3329 _]
                      tunnel: [w3329 1.0] -> w3324
                      frame False {
                        n2840 = local write "Cycles elapsed"(w3329) -> ()
                      }
                      frame True {
                      }
                    }
                    n2841 = Greater?(x=w3318, y=w3317) -> (0:w3326:bool)
                    n2842 = Subtract(x=w3317, y=w3318) -> (x-y=w3316:dbl)
                    n2843 = Multiply(x=w3316, y=60.0) -> (x*y=w3315:dbl)
                    n2844 = local write "Time Remaining"(w3315) -> ()
                    n2845 = local write "Remaining Time"(w3315) -> ()
                    n2846 = case shown="True" w3326 {
                      frame False {
                      }
                      frame True {
                        n2847 = stacked-sequence {
                          frame #0 {
                            w3334 = T19."Enabled" ("Disabled")
                            w3333 = FALSE ("TEST FILE NAM,E SAVED")
                            w3335 = "" ("FILE")
                            w3336 = TRUE ("Visible")
                            n2848 = local write "Humidity"(FALSE ("Humidity")) -> ()
                            n2849 = local write "RUN"(FALSE ("OK Button 2")) -> ()
                            n2850 = local write "Heater Button"(FALSE ("Heater Button")) -> ()
                            n2851 = local write "Auto Start Test"(FALSE ("Auto Start Test")) -> ()
                            n2852 = local write "TestCompFlg"(TRUE ("StpFlg")) -> ()
                            n2853 = local read "Humidity ( %RH )"() -> (→"Rh After":dbl)
                            n2854 = property on="STOP 2" class="Bool (strict)"("Disabled"=u8 0) -> ()  [unwired: 2 in, 2 out]
                            n2855 = local read "EVENT LOG"() -> (w3341:string)
                            n2856 = call "Event Log.vi"("Content"="Test Completed", "EVENT LOG"=w3341) -> ("EVENT LOG"=w3340:string)  [unwired: 8 in, 1 out]
                            n2857 = property on="RUN" class="Bool (strict)"("Visible"=w3336) -> ()  [unwired: 2 in, 2 out]
                            n2858 = property on="Auto Start Test" class="Bool (strict)"("Visible"=w3336) -> ()  [unwired: 2 in, 2 out]
                            n2859 = local write "Batch Ref Num :"(w3335) -> ()
                            n2860 = local write "FILE"(w3335) -> ()
                            n2861 = local write "EVENT LOG"(w3340) -> ()
                            n2862 = local write "TEST FILE NAM,E SAVED"(w3333) -> ()
                            n2863 = local write "Fuel Discription :"(w3335) -> ()
                            n2864 = local write "START TEMP"(w3333) -> ()
                            n2865 = local write "Remarks :"(w3335) -> ()
                            n2866 = local write "Main Dashboard Buttons"(T1."Imaging" ("Main Dashboard Buttons")) -> ()
                            n2867 = local write "Main Tab"(T4."Adv Scar" ("Main Tab")) -> ()
                            n2868 = property on="FRICVALZ 2" class="Bool (strict)"("DisabledEnum"=w3334) -> ()  [unwired: 2 in, 2 out]
                            n2869 = property on="FRICVALZ 3" class="Bool (strict)"("DisabledEnum"=w3334) -> ()  [unwired: 2 in, 2 out]
                            n2870 = property on="FRICVALZ 4" class="Bool (strict)"("DisabledEnum"=w3334) -> ()  [unwired: 2 in, 2 out]
                          }
                          frame #1 {
                            n2871 = Wait (ms)(milliseconds to wait=u32 2000) -> ()  [unwired: 1 out]
                          }
                          frame #2 {
                            n2872 = local write "Due Write"("VC;0") -> ()
                          }
                          frame #3 {
                            n2873 = Wait (ms)(milliseconds to wait=u32 2000) -> ()  [unwired: 1 out]
                          }
                          frame #4 {
                            n2874 = local write "Due Write"("VC;0") -> ()
                          }
                          frame #5 {
                            n2875 = Wait (ms)(milliseconds to wait=u32 2000) -> ()  [unwired: 1 out]
                          }
                          frame #6 {
                            n2876 = local write "Due Write"("ST;0") -> ()
                          }
                          frame #7 {
                            n2877 = local write "measured_stroke"(0.0 ("measured_stroke")) -> ()
                            n2878 = Wait (ms)(milliseconds to wait=u32 1500) -> ()  [unwired: 1 out]
                          }
                          frame #8 {
                            n2879 = local write "Due Write"("HE;0") -> ()
                            n2880 = local write "Humidity 2"(TRUE ("Humidity")) -> ()
                          }
                        }
                      }
                    }
                    n2881 = Divide(x=w3318, y=w3317) -> (x/y=w3321:dbl)
                    n2882 = Multiply(x=w3321, y=100.0) -> (x*y=w3319:dbl)
                    n2883 = local write "Test Duration Status"(w3319) -> ()
                  }
                }
              }
              frame #2 {
                n2884 = case shown="True" "Heater Button" {
                  tunnel: [0.0 ("output") w3456] -> w3434
                  frame False {
                    w3437 = TRUE ("tmpchk")
                    n2885 = local read "TEMP"() -> (w3438:dbl)
                    n2886 = local write "Temp ini"(w3438) -> ()
                    n2887 = local write "Reset 4"(w3437) -> ()
                    n2888 = local write "tmpchk"(w3437) -> ()
                    n2889 = local write "reinit"(TRUE ("reinit")) -> ()
                    n2890 = local write "manual temp log"(TRUE ("manual temp log")) -> ()
                  }
                  frame True {
                    # "Logic to turn off\nthe heater when \ntemp is not rising.\nTime - 60 sec\nDelta t- 5°c"
                    n2891 = local read "Temp ini"() -> (w3445:dbl)
                    n2892 = local read "Auto Start Test"() -> (w3441:bool)
                    n2893 = Less?(x=w3445, y=53.0) -> (x < y?=w3443:bool)
                    n2894 = case shown="False" w3441 {
                      frame False {
                        n2895 = local read "Set Temp"() -> (w3465:dbl)
                        n2896 = local read "TEMP"() -> (w3464:dbl)
                        n2897 = Subtract(x=w3465, y=w3464) -> (x-y=w3463:dbl)
                        n2898 = Absolute Value(x=w3463) -> (abs(x)=w3462:dbl)
                        n2899 = Less?(x=w3462, y=0.5) -> (x < y?=w3460:bool)
                        n2900 = case shown="True" w3460 {
                          tunnel: "manual temp log" -> [_ w3466]
                          frame False {
                          }
                          frame True {
                            n2901 = case shown="True" w3466 {
                              selector: w3466 -> [_ w3467]
                              frame False {
                              }
                              frame True {
                                # "#Event log"
                                n2902 = Not(x=w3467) -> (.not. x?=w3468:bool)
                                n2903 = local write "manual temp log"(w3468) -> ()
                                n2904 = local read "EVENT LOG"() -> (w3471:string)
                                n2905 = call "Event Log.vi"("Content"="Target Temperature reached", "EVENT LOG"=w3471) -> ("EVENT LOG"=w3470:string)  [unwired: 8 in, 1 out]
                                n2906 = local write "EVENT LOG"(w3470) -> ()
                              }
                            }
                          }
                        }
                      }
                      frame True {
                        n2907 = local write "manual temp log"(TRUE ("manual temp log")) -> ()
                      }
                    }
                    n2908 = And(x="tmpchk", y=w3443) -> (x .and. y?=w3446:bool)
                    n2909 = case shown="True" w3446 {
                      frame False {
                      }
                      frame True {
                        n2910 = call "Elapsed Time8"("Time Target (s)"=300.0, "Reset"="Reset 4") -> ("Time has Elapsed"=w3473:bool)  [unwired: 10 in, 7 out]
                        n2911 = flat-sequence {
                          tunnel: w3473 -> [_]
                          frame #0 {
                            n2912 = local write "Reset 4"(FALSE ("Reset 4")) -> ()
                          }
                        }
                        n2913 = case shown="True" w3473 {
                          frame False {
                          }
                          frame True {
                            n2914 = local read "Temp ini"() -> (w3480:dbl)
                            n2915 = Add(x=w3480, y=5.0) -> (x+y=w3478:dbl)
                            n2916 = local read "TEMP"() -> (w3481:dbl)
                            n2917 = Greater?(x=w3481, y=w3478) -> (0:w3479:bool)
                            n2918 = case shown="False" w3479 {
                              frame False {
                                n2919 = local write "Heater Button"(FALSE ("Heater Button")) -> ()
                              }
                              frame True {
                                n2920 = local write "tmpchk"(FALSE ("tmpchk")) -> ()
                              }
                            }
                          }
                        }
                      }
                    }
                    n2921 = local read "Set Temp"() -> (w3454:dbl)
                    n2922 = local read "TEMP"() -> (w3448:dbl)
                    n2923 = call-poly <vilib>:"PID.vi"("reinitialize? (F)"="reinit", "dt (s)"=-1.0, "process variable"=w3448, "setpoint"=w3454) -> ("output"=w3451:dbl)  [unwired: 6 in, 1 out]
                    n2924 = Subtract(x=w3454, y=w3448) -> (x-y=w3455:dbl)
                    n2925 = Add(x=w3454, y=0.5) -> (x+y=w3452:dbl)
                    n2926 = Greater Or Equal?(x=w3448, y=w3452) -> ()  [unwired: 1 out]
                    n2927 = Select(t=0.0, s=FALSE, f=w3451) -> (s? t:f=w3450:dbl)
                    "PID output" <- w3450
                    n2928 = flat-sequence {
                      tunnel: w3450 -> [w3484]
                      tunnel: [w3484] -> w3456
                      frame #0 {
                        n2929 = local write "reinit"(FALSE ("reinit")) -> ()
                      }
                    }
                    n2930 = Bundle(w3455, "output"=w3450, "TEMP"=w3448) -> ()  [unwired: 1 in, 1 out]
                  }
                }
                "PID-out" <- w3434
              }
              frame #3 {
                n2931 = local read "TEMP"() -> (w3486:dbl)
                n2932 = Greater Or Equal?(x=w3486, y="Set Temp 2") -> (x >= y?=w3491:bool)
                n2933 = case shown="True" w3491 {
                  tunnel: [FALSE TRUE] -> w3489
                  frame False {
                  }
                  frame True {
                  }
                }
                "Status 13" <- w3489
                n2934 = And(x=w3489, y="trip1 8") -> (x .and. y?=w3488:bool)
                n2935 = case shown="True" w3488 {
                  frame False {
                    n2936 = local write "Heater Trip Temp"(TRUE ("Heater Trip Temp")) -> ()
                  }
                  frame True {
                    w3494 = FALSE ("OK Button 2")
                    n2937 = case shown="True" "Heater Trip Temp" {
                      selector: "Heater Trip Temp" -> [_ w3496]
                      frame False {
                      }
                      frame True {
                        n2938 = Not(x=w3496) -> (.not. x?=w3495:bool)
                        n2939 = local read "EVENT LOG"() -> (w3499:string)
                        n2940 = local write "Heater Trip Temp"(w3495) -> ()
                        n2941 = call "Event Log.vi"("Content"="Heater Trip", "EVENT LOG"=w3499) -> ("EVENT LOG"=w3498:string)  [unwired: 8 in, 1 out]
                        n2942 = local write "EVENT LOG"(w3498) -> ()
                      }
                    }
                    n2943 = local write "RUN"(w3494) -> ()
                    n2944 = property on="Auto Start Test" class="Bool (strict)"("Value"=w3494) -> ()  [unwired: 2 in, 2 out]
                    n2945 = local write "Heater Button"(w3494) -> ()
                  }
                }
              }
            }
